vi "dfd_FXP MRate FIR Simu.vi"(6 "output phase":i32, 7 "init? (T)":bool, 8 "FXPMRateSimState in":T1, 10 "multirate filter":T3={"mMRate_Structure"=enum."CIC", "mMRate_Mode"=0, "mMRate_Factor"=0, "mMRate_FIRParams"={"mMRate_FIR_H"=[], "mMRate_FIR_IsNyquist?"=FALSE, "mMRate_FIR_IsSymmetric?"=FALSE}, "mMRate_CICParams"={"mMRate_CIC_#Stage"=2, "mMRate_CIC_Lag"=1, "mMRate_CIC_Type"=enum."Lowpass"}, "mMRate_Order"=0, "mMRate_Version"="2.0", "mMRate_Comments"="", "mMRate_RationalFactor"={"mMRate_L"=-1, "mMRate_M"=-1}, "mMRate_Fs"=0.0, "mMRate_Quantized?"=FALSE, "mMRate_QFilterGain"=1.0, "mMRate_CoefWl"=16, "mMRate_Scaling"={"mMRate_ScaleByPowerOf2?"=FALSE, "mMRate_ScaleType"=enum."Time Domain 1-Norm"}, "mMRate_InputWl"=16, "mMRate_OutputWl"=16, "mMRate_OutputMode"=enum."Truncation", "mMRate_MultMode"=enum."Truncated", "mMRate_BitPruning"=FALSE, "mMRate_GainWl"=16, "mMRate_OutputFwl"=0, "mMRate_SumIwl"=0, "mMRate_InputIwl "=16, "mMRate_SumWl"=32, "mMRate_CoefIwl"=0} {"mMRate_SumWl" min=1 max=32 step=1; "mMRate_InputIwl" min=1 max=32 step=1; "mMRate_GainWl" min=1 max=32 step=1; "mMRate_OutputWl" min=1 max=32 step=1; "mMRate_InputWl" min=1 max=32 step=1; "mMRate_CoefWl" min=1 max=32 step=1; "mMRate_Mode" items=["Default"=-1, "No Rate Change"=0, "Interpolation"=1, "Decimation"=2, "Interpolated"=3, "Rational"=4]}, 11 "signal in":i32[](array[numeric])) -> (0 "FXPMRateSimState out":T1, 3 "signal out":i32[](array[numeric]))   [LabVIEW 2017, in "NI_DigFilter_FXP.lvlib"]
uses:
  <vilib>/addons/Digital Filter Design/NI_DigFilter_FXP.lvlib
  <vilib>/addons/Digital Filter Design/_Objects.llb/DFD Multirate Filter Obj.ctl
  <vilib>/addons/Digital Filter Design/_Objects.llb/DFD Multirate Mode.ctl
  <vilib>/addons/Digital Filter Design/_Objects.llb/DFD Coef Norm Type.ctl
  <vilib>/addons/Digital Filter Design/_Objects.llb/DFD Round-off Mode.ctl
  <vilib>/addons/Digital Filter Design/_Objects.llb/DFD FXP MRate Multiply Mode.ctl
  <vilib>/addons/Digital Filter Design/_Objects.llb/dfd_FXP MRate Simu State.ctl
  <vilib>/addons/Digital Filter Design/_Objects.llb/dfd_Integer I160.ctl
  <vilib>/addons/Digital Filter Design/NI_DigFilterLicensed.lvlib
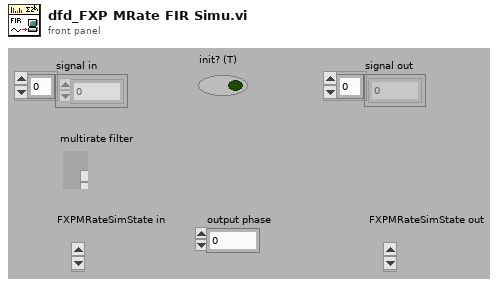
[diagram p1: front panel]
types:
  T1 = typedef "dfd_FXP MRate Simu State.ctl" = cluster{"acc1":T2[], "acc2":T2[], "FIR state":i64[], "next phase":i32}
  T2 = typedef "dfd_Integer I160.ctl" = cluster{"Hi [I32]":i32, "Lo3 [U32]":u32, "Lo2 [U32]":u32, "Lo1 [U32]":u32, "Lo0 [U32]":u32}
  T3 = typedef "NI_DigFilterLicensed.lvlib/DFD Multirate Filter Obj.ctl" = cluster{"mMRate_Structure":enum16{"CIC", "FIR", "IIR", "Lattice"}, "mMRate_Mode":T4, "mMRate_Factor":i32, "mMRate_FIRParams":cluster{"mMRate_FIR_H":dbl[], "mMRate_FIR_IsNyquist?":bool, "mMRate_FIR_IsSymmetric?":bool}, "mMRate_CICParams":cluster{"mMRate_CIC_#Stage":i32, "mMRate_CIC_Lag":i32, "mMRate_CIC_Type":enum16{"Lowpass", "Highpass"}}, "mMRate_Order":i32, "mMRate_Version":string, "mMRate_Comments":string, "mMRate_RationalFactor":cluster{"mMRate_L":i32, "mMRate_M":i32}, "mMRate_Fs":dbl, "mMRate_Quantized?":bool, "mMRate_QFilterGain":dbl, "mMRate_CoefWl":i16, "mMRate_Scaling":cluster{"mMRate_ScaleByPowerOf2?":bool, "mMRate_ScaleType":T5}, "mMRate_InputWl":i16, "mMRate_OutputWl":i16, "mMRate_OutputMode":T6, "mMRate_MultMode":T7, "mMRate_BitPruning":bool, "mMRate_GainWl":i16, "mMRate_OutputFwl":i16, "mMRate_SumIwl":i16, "mMRate_InputIwl ":i16, "mMRate_SumWl":i16, "mMRate_CoefIwl":i16}
  T4 = typedef "NI_DigFilterLicensed.lvlib/DFD Multirate Mode.ctl" = i16
  T5 = typedef "NI_DigFilterLicensed.lvlib/DFD Coef Norm Type.ctl" = enum16{"No Norm", "Time Domain 1-Norm", "Time Domain 2-Norm", "Time Domain Inf-Norm"}
  T6 = typedef "NI_DigFilterLicensed.lvlib/DFD Round-off Mode.ctl" = enum16{"Nearest", "Truncation"}
  T7 = typedef "NI_DigFilterLicensed.lvlib/DFD FXP MRate Multiply Mode.ctl" = enum16{"Truncated", "Full"}
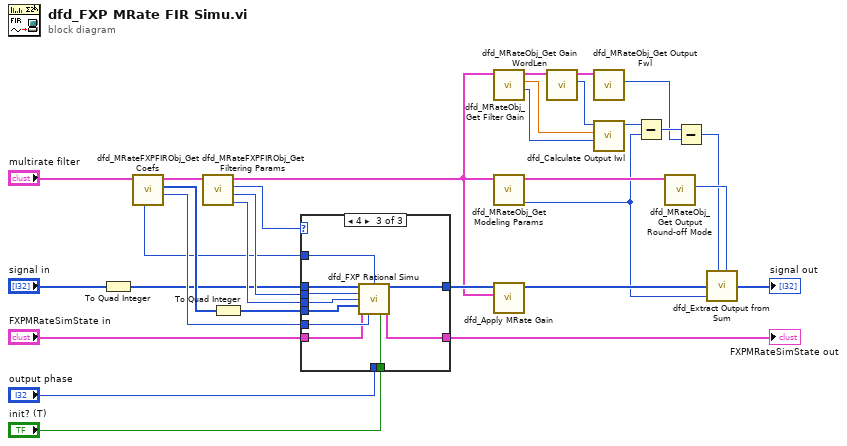
[diagram p0: block diagram]
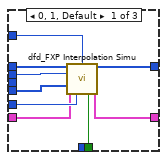
[diagram p2: hidden frame]
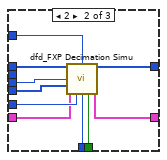
[diagram p3: hidden frame]
diagram:
  n1 = To Quad Integer(1:"signal in") -> (0:w14:i64[])
  n2 = call <vilib>:"dfd_MRateFXPFIRObj_Get Coefs.vi"("FXP MRate FIR in"="multirate filter") -> ("#taps per phase"=w26:i32, "coef"=w27:i32[], "dup FXP MRate FIR"=w30:T3, "PROD2SUM"=w15:i16)  [unwired: 7 out]
  n3 = call <vilib>:"dfd_MRateFXPFIRObj_Get Filtering Params.vi"("FXP MRate FIR in"=w30) -> ("M"=w28:i32, "L"=w29:i32, "mode"=w25:T4, "dup FXP MRate FIR"=w6:T3)  [unwired: 7 out]
  n4 = To Quad Integer(1:w27) -> (0:w13:i64[])
  n5 = case shown="4" w25 {
    tunnel: [w39 w49 w59] -> w23
    tunnel: w14 -> [w40 w50 w60]
    tunnel: "output phase" -> [_ w48 _]
    tunnel: w29 -> [w38 _ w51]
    tunnel: w28 -> [_ w43 w58]
    tunnel: w13 -> [w37 w47 w53]
    tunnel: w26 -> [w36 w46 w57]
    tunnel: w15 -> [w35 w45 w56]
    tunnel: "init? (T)" -> [w34 w44 w55]
    tunnel: "FXPMRateSimState in" -> [w33 w42 w54]
    tunnel: [w32 w41 w52] -> w17
    frame 0, 1, Default {
      n6 = call <vilib>:"dfd_FXP Interpolation Simu.vi"("signal in"=w40, "PROD2SUM"=w35, "init?"=w34, "interpolation factor"=w38, "coef"=w37, "FXPMRateSimState in"=w33, "#taps per phase"=w36) -> ("signal out"=w39:i64[], "FXPMRateSimState out"=w32:T1)  [unwired: 1 in, 6 out]
    }
    frame 2 {
      n7 = call <vilib>:"dfd_FXP Decimation Simu.vi"("signal in"=w50, "PROD2SUM"=w45, "init?"=w44, "decimation factor"=w43, "coef"=w47, "FXPMRateSimState in"=w42, "#taps per phase"=w46, "output phase"=w48) -> ("signal out"=w49:i64[], "FXPMRateSimState out"=w41:T1)  [unwired: 2 in, 4 out]
    }
    frame 4 {
      n8 = call <vilib>:"dfd_FXP Rational Simu.vi"("signal in"=w60, "PROD2SUM"=w56, "init?"=w55, "L"=w51, "M"=w58, "coef"=w53, "FXPMRateSimState in"=w54, "#taps per phase"=w57) -> ("signal out"=w59:i64[], "FXPMRateSimState out"=w52:T1)  [unwired: 1 in, 5 out]
    }
  }
  "FXPMRateSimState out" <- w17
  n9 = call <vilib>:"dfd_MRateObj_Get Filter Gain.vi"("multirate filter in"=w6) -> ("sum iwl"=w9:i16, "gain"=w10:dbl, "dup multirate filter"=w11:T3)  [unwired: 8 out]
  n10 = call <vilib>:"dfd_MRateObj_Get Modeling Params.vi"("multirate filter in"=w6) -> ("output wl"=w4:i16, "dup multirate filter"=w21:T3)  [unwired: 9 out]
  n11 = call <vilib>:"dfd_Apply MRate Gain.vi"("multirate filter"=w6, "signal in"=w23) -> ("signal out"=w22:i64[])  [unwired: 9 out]
  n12 = call <vilib>:"dfd_MRateObj_Get Gain WordLen.vi"("multirate filter in"=w11) -> ("gain wl"=w7:i16, "dup multirate filter"=w5:T3)  [unwired: 9 out]
  n13 = call <vilib>:"dfd_MRateObj_Get Output Fwl.vi"("multirate filter in"=w5) -> ("output fwl"=w2:i16)  [unwired: 9 in, 1 out]
  n14 = call <vilib>:"dfd_Calculate Output Iwl.vi"("sum iwl"=w9, "gain value"=w10, "gain wl"=w7) -> ("output iwl"=w8:i16)  [unwired: 8 out]
  n15 = Subtract(x=w8, y=w4) -> (x-y=w3:i16)
  n16 = call <vilib>:"dfd_MRateObj_Get Output Round-off Mode.vi"("multirate filter in"=w21) -> ("output round-off mode"=w20:T6)  [unwired: 10 out]
  n17 = Subtract(x=w3, y=w2) -> (x-y=w1:i16)
  n18 = call <vilib>:"dfd_Extract Output from Sum.vi"("output iwl diff"=w1, "x"=w22, "output wl"=w4, "q_mode"=w20) -> ("y"=→"signal out":i32[])  [unwired: 5 out]
